vi "GUI_GlassmanEK40R15_VI.vi"() -> ()   [LabVIEW 2013]
uses:
  Shared/GUI_Template/GUI_master/tcp_new_data_event.ctl
  Shared/GUI_Template/GUI_master/tcp new data cluster.ctl
panel:
  out "tcp data event":T1
  in  "Refresh Button":bool
  in  "Select device":string(combo)="PL1-PresCtl"
  in  "stop":bool
  in  "enable::1":enum16{"off", "on", "reset", "fault"}(ring) caption="Enable HV"
  in  "voltage::1":dbl caption="Voltage (KV)" min=0.0 max=40.0
  out "voltageMode::1":enum16{"off", "on"}(ring) caption="Voltage Mode"
  in  "GUIdevice 1":string="PL1-GlassmanHV"
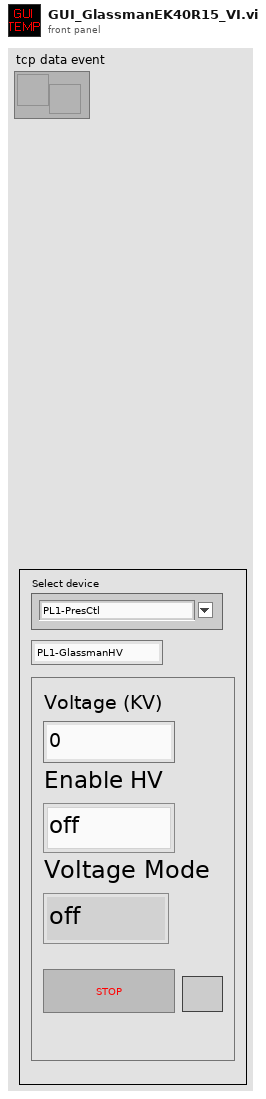
[diagram p1: front panel]
types:
  T1 = typedef "tcp_new_data_event.ctl" = refnum<user-event>
  T2 = enum32{"invalid app kind", "Development System", "Run Time System", "Student Edition", "Embedded LabVIEW", "Evaluation", "Custom"}
  T3 = typedef "tcp new data cluster.ctl" = cluster{"EventEnum":enum16{"new data", "connection status update"}, "Device name":string}
  T4 = enum32{"Invalid", "Standard", "Closed", "Hidden", "Minimized", "Maximized"}
  T5 = cluster{"Core":cluster{"Current VI Reference":refnum<vi>, "Close Panel on Exit?":bool}, "Your Boolean data":bool, "Your string data":string, "SuperGUI":cluster{"STOP queue":refnum<queue>, "SuperGUI ref":refnum<vi>}}
  T6 = cluster{"STOP queue":refnum<queue>, "SuperGUI ref":refnum<vi>}
  T7 = cluster{"Current VI Reference":refnum<vi>, "Close Panel on Exit?":bool}
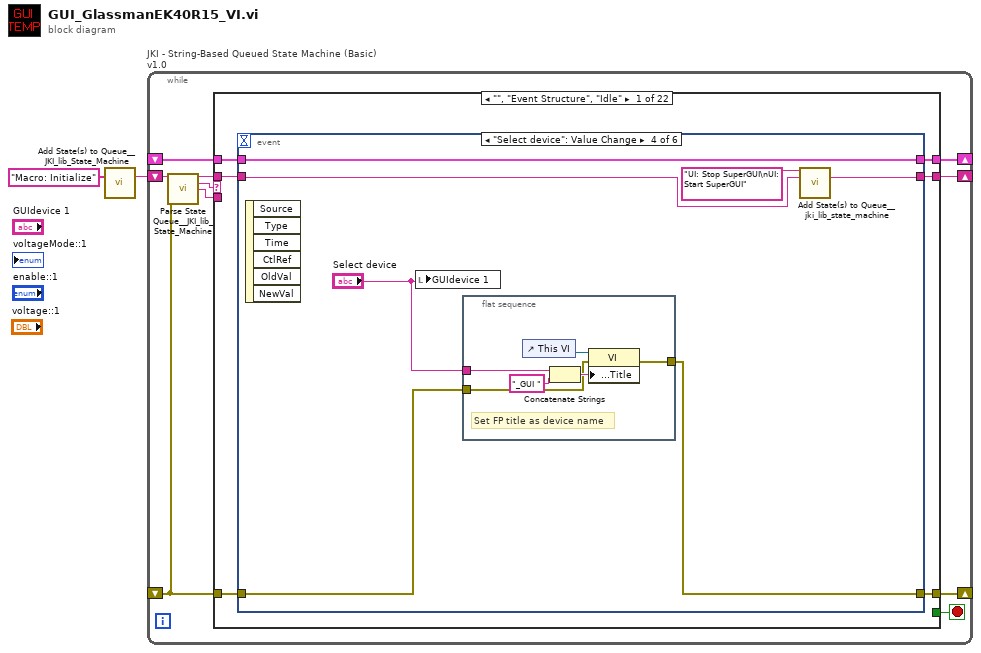
[diagram p0: block diagram]
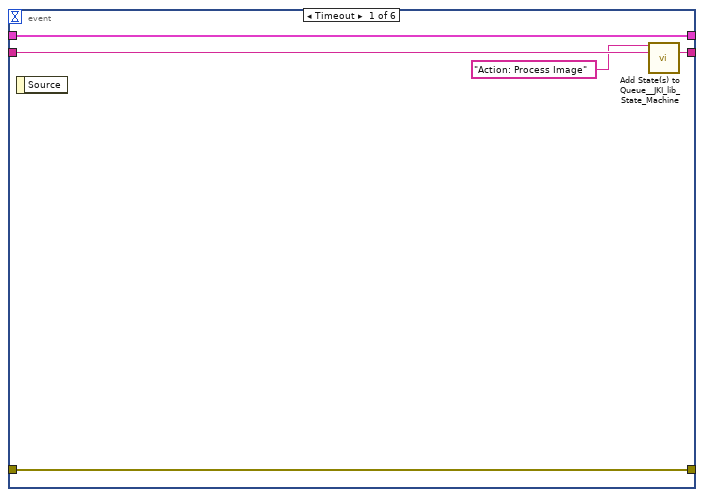
[diagram p2: hidden frame]
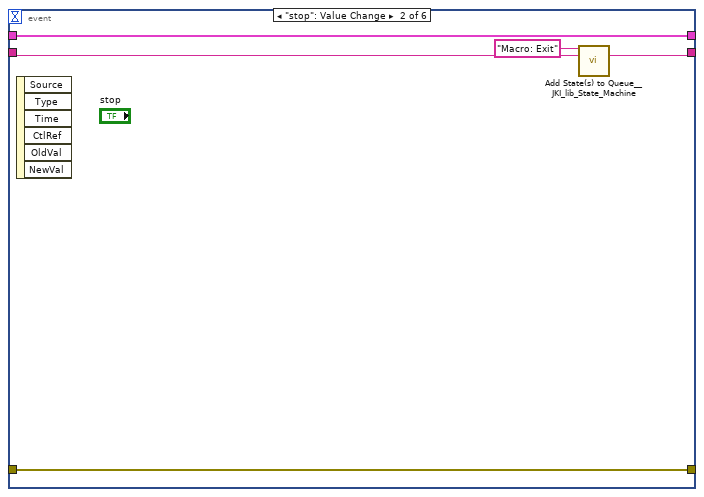
[diagram p3: hidden frame]
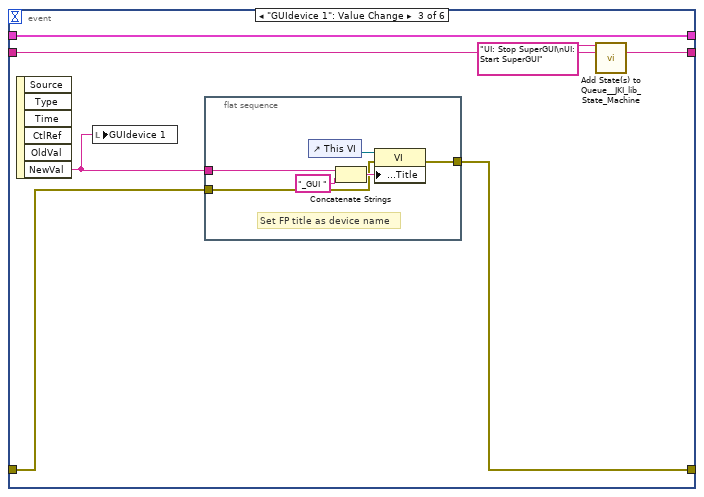
[diagram p4: hidden frame]
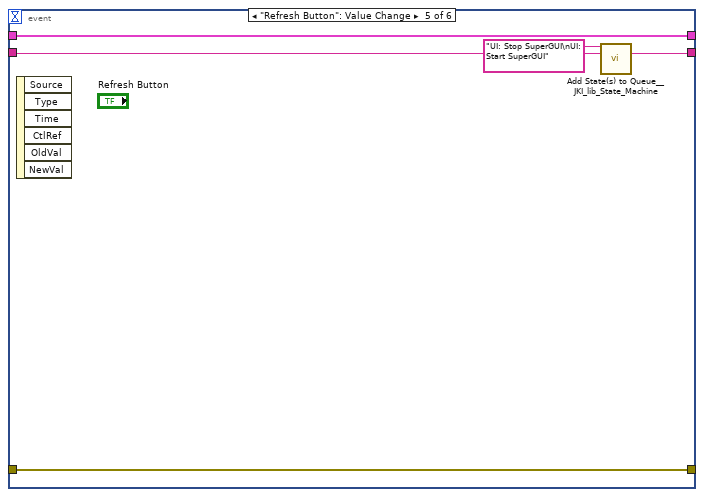
[diagram p5: hidden frame]
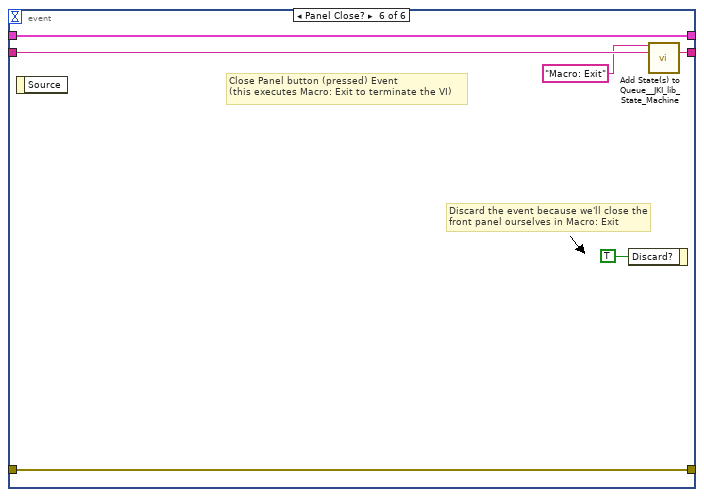
[diagram p6: hidden frame]
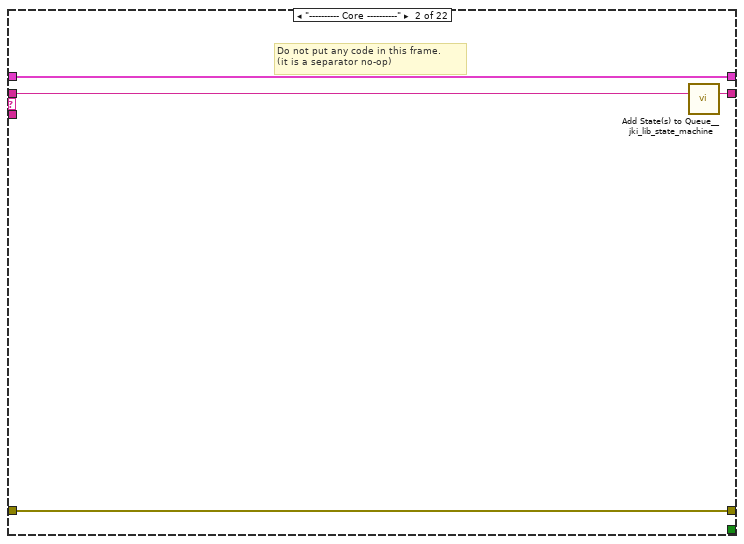
[diagram p7: hidden frame]
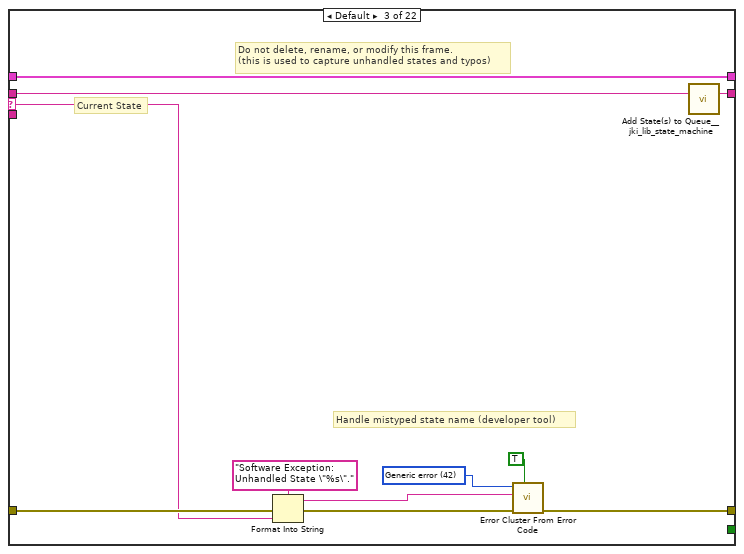
[diagram p8: hidden frame]
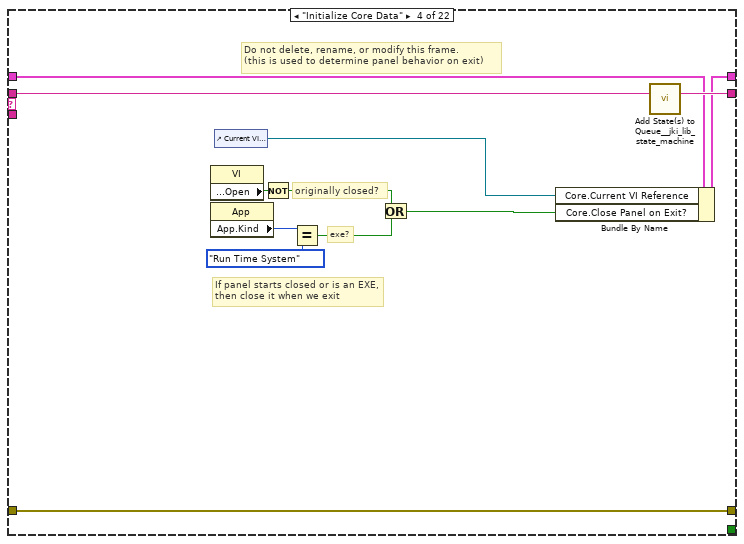
[diagram p9: hidden frame]
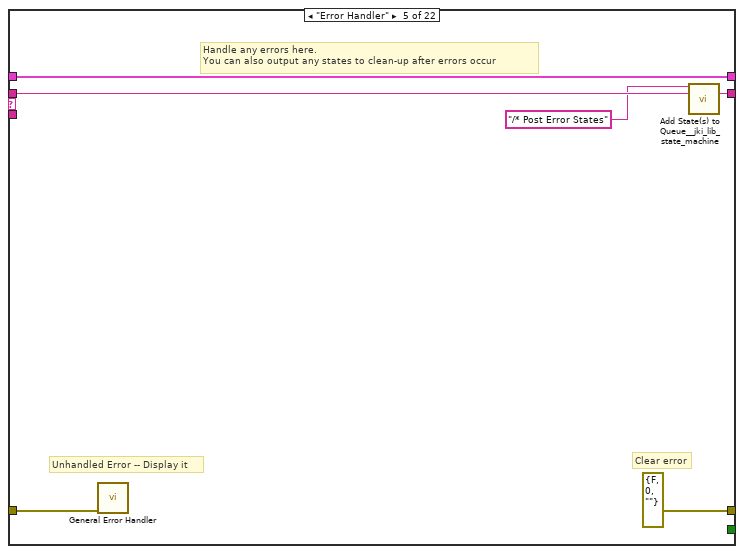
[diagram p10: hidden frame]
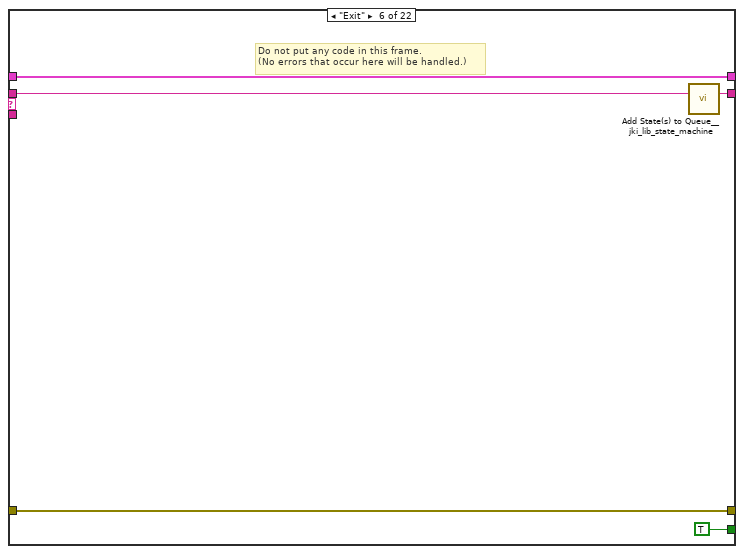
[diagram p11: hidden frame]
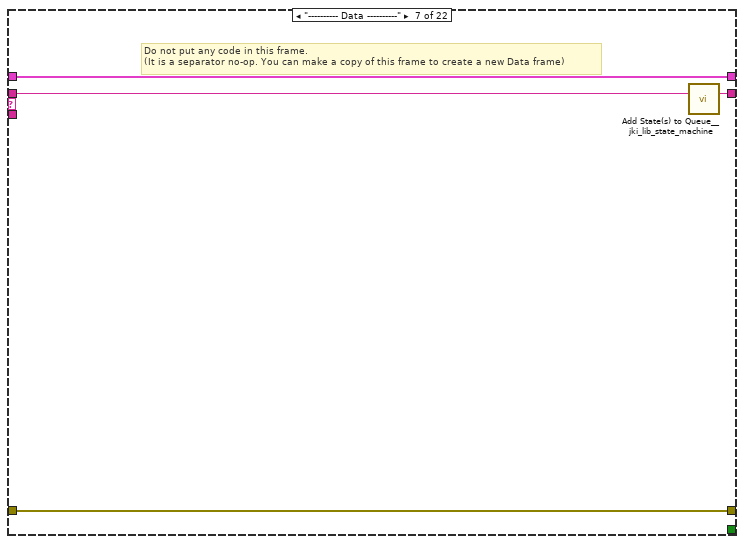
[diagram p12: hidden frame]
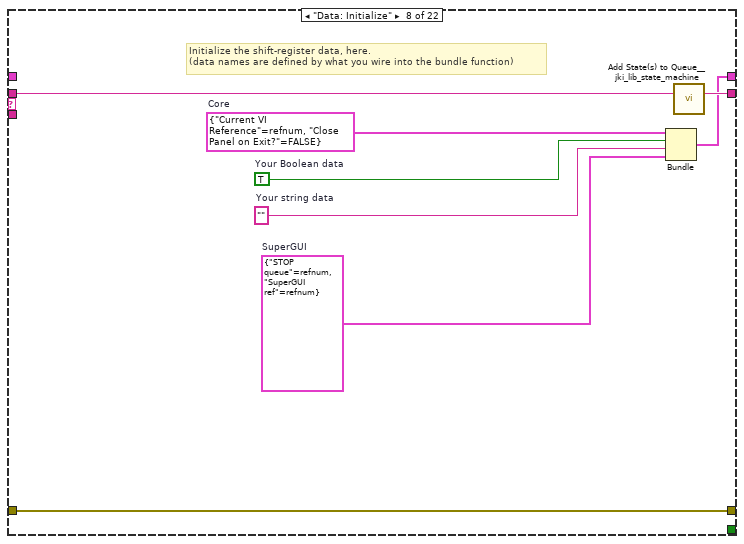
[diagram p13: hidden frame]
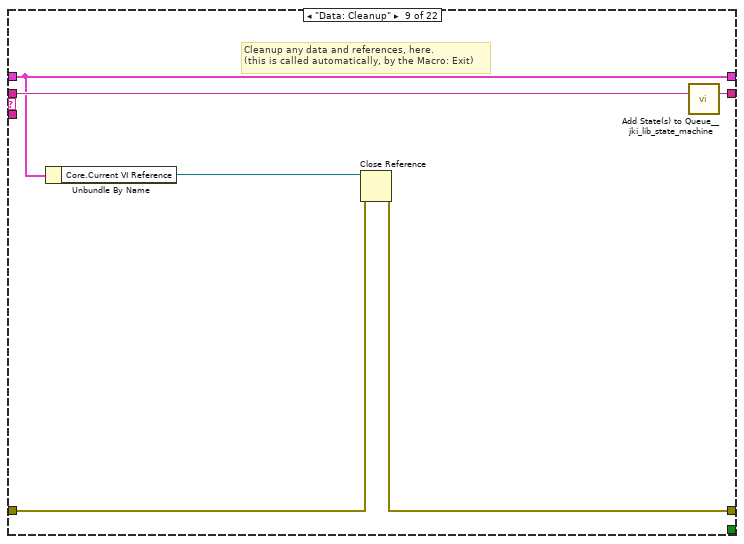
[diagram p14: hidden frame]
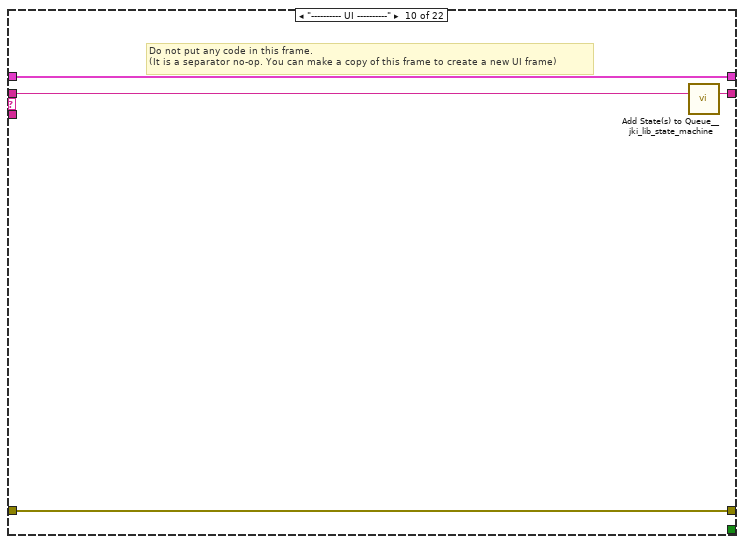
[diagram p15: hidden frame]
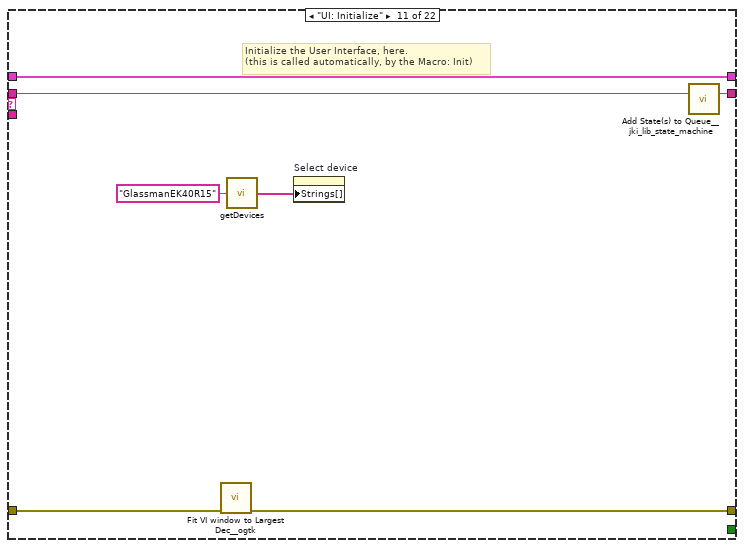
[diagram p16: hidden frame]
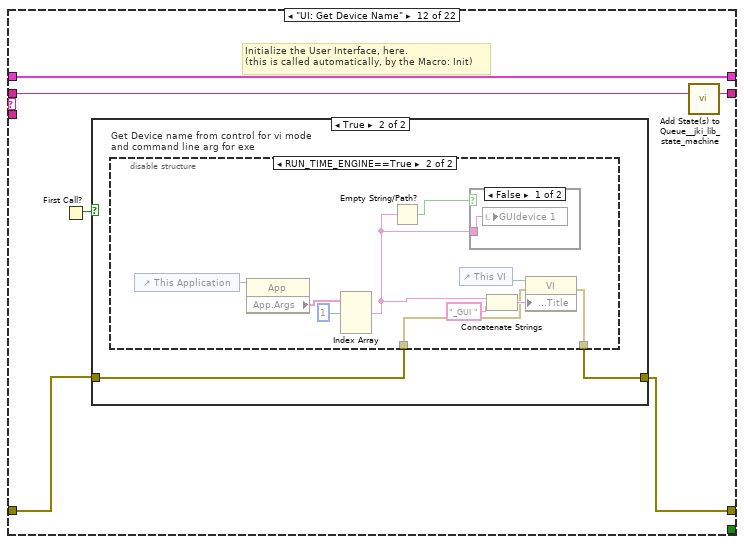
[diagram p17: hidden frame]
diagram:
  n1 = call <vilib>:"Add State(s) to Queue__JKI_lib_State_Machine.vi"("State(s) in (\"\")"="Macro: Initialize") -> ("States Out"=w2:string)  [unwired: 14 in]
  n2 = while "JKI - String-Based Queued State Machine (Basic) v1.0" {
    shift-right: [w5] -> _
    shift-left: _ -> [w4]
    shift-right: [w8] -> _
    shift-left: _ -> [w3]
    shift-right: [w7] -> _
    shift-left: w2 -> [w9]
    stop <- w6 stop-if-true
    n3 = call <vilib>:"Parse State Queue__JKI_lib_State_Machine.vi"("State Queue"=w9, "Error In (no error)"=w3) -> ("Remaining States"=w11:string, "Current State"=w12:string, "Arguments"=w10:string)  [unwired: 11 in]
    n4 = case shown="\"\", \"Event Structure\", \"Idle\"" w12 {
      selector: w12 -> [_ _ w70 _ _ _ _ _ _ _ _ _ _ _ _ _ _ _ _ _ _ _]
      tunnel: w11 -> [w18 w69 w74 w92 w98 w103 w107 w115 w121 w125 w132 w138 w173 w181 w187 w198 w224 w229 w239 w243 w247 w251]
      tunnel: w10 -> [_ _ _ _ _ _ _ _ _ _ _ _ _ _ w182 w192 _ _ _ _ _ _]
      tunnel: w4 -> [w16 w66 w72 w83 w95 w101 w104 _ w116 w122 w130 w136 w164 w176 w185 w194 w221 w226 w236 w240 w244 w248]
      tunnel: [w15 w67 w76 w89 errorcluster {"status"=FALSE, "code"=0, "source"=""} ("error out") w100 w105 w112 w117 w123 w128 w133 w157 w174 w183 w195 w222 w227 w237 w241 w245 w249] -> w8
      tunnel: w3 -> [w14 w67 w75 w89 w94 w100 w105 w112 w118 w123 w129 w134 w158 w175 w184 w196 w222 w227 w237 w241 w245 w249]
      tunnel: [w17 w68 w73 w91 w97 w102 w106 w114 w120 w124 w131 w137 w172 w180 w186 w197 w223 w228 w238 w242 w246 w250] -> w7
      tunnel: [_ _ _ _ _ TRUE _ _ _ _ _ _ _ _ _ _ _ _ _ _ _ _] -> w6
      tunnel: [w13 w66 w72 w90 w95 w101 w104 w113 w116 w122 w130 w136 w163 w176 w185 w194 w221 w226 w236 w240 w244 w248] -> w5
      frame "", "Event Structure", "Idle" {
        n5 = event shown="[3] \"Select device\": Value Change" {
          selector: _ -> [_ _ _ _ _ _]
          dyn-events: _ -> [_ _ _ _ _ _]
          timeout: _ -> [_ _ _ _ _ _]
          tunnel: w18 -> [w23 w26 w32 w43 w57 w65]
          tunnel: [w22 w25 w31 w42 w56 w64] -> w17
          tunnel: w16 -> [w20 w28 w35 w48 w59 w62]
          tunnel: [w21 w27 w33 w45 w58 w63] -> w15
          tunnel: w14 -> [w21 w27 w34 w46 w58 w63]
          tunnel: [w20 w28 w35 w48 w59 w62] -> w13
          event Timeout {
            n6 = event-data() -> ()  [unwired: 1 in, 1 out]
            n7 = call <vilib>:"Add State(s) to Queue__JKI_lib_State_Machine.vi"("State(s) in Front (\"\")"="Action: Process Image" ("State(s) in Front (\"\")"), "State(s) in (\"\")"=w23) -> ("States Out"=w22:string)  [unwired: 13 in]
          }
          event "stop": Value Change {
            n8 = event-data() -> ()  [unwired: 1 in, 6 out]
            n9 = call <vilib>:"Add State(s) to Queue__JKI_lib_State_Machine.vi"("State(s) in Front (\"\")"="Macro: Exit", "State(s) in (\"\")"=w26) -> ("States Out"=w25:string)  [unwired: 13 in]
          }
          event "GUIdevice 1": Value Change {
            n10 = event-data() -> ("NewVal"=w29:string)  [unwired: 1 in, 5 out]
            n11 = local write "GUIdevice 1"(w29) -> ()
            n12 = flat-sequence {
              tunnel: [w38] -> w33
              tunnel: w34 -> [w37]
              tunnel: w29 -> [w36]
              frame #0 {
                # "Set FP title as device name"
                n13 = control-ref of="This VI"() -> (w41:refnum<vi>)
                n14 = Concatenate Strings(w36, "_GUI ") -> (w40:string)
                n15 = property class="VI"(reference=w41, error in=w37, "Front Panel.Title"=w40) -> (error out=w38:errorcluster)  [unwired: 1 out]
              }
            }
            n16 = call <vilib>:"Add State(s) to Queue__JKI_lib_State_Machine.vi"("State(s) in Front (\"\")"="UI: Stop SuperGUI\nUI: Start SuperGUI", "State(s) in (\"\")"=w32) -> ("States Out"=w31:string)  [unwired: 13 in]
          }
          event "Select device": Value Change {
            n17 = event-data() -> ()  [unwired: 1 in, 6 out]
            n18 = local write "GUIdevice 1"("Select device") -> ()
            n19 = flat-sequence {
              tunnel: [w51] -> w45
              tunnel: w46 -> [w50]
              tunnel: "Select device" -> [w49]
              frame #0 {
                # "Set FP title as device name"
                n20 = control-ref of="This VI"() -> (w54:refnum<vi>)
                n21 = Concatenate Strings(w49, "_GUI ") -> (w53:string)
                n22 = property class="VI"(reference=w54, error in=w50, "Front Panel.Title"=w53) -> (error out=w51:errorcluster)  [unwired: 1 out]
              }
            }
            n23 = call <vilib>:"Add State(s) to Queue__jki_lib_state_machine.vi"("State(s) in Front (\"\")"="UI: Stop SuperGUI\nUI: Start SuperGUI", "State(s) in (\"\")"=w43) -> ("States Out"=w42:string)  [unwired: 13 in]
          }
          event "Refresh Button": Value Change {
            n24 = event-data() -> ()  [unwired: 1 in, 6 out]
            n25 = call <vilib>:"Add State(s) to Queue__JKI_lib_State_Machine.vi"("State(s) in Front (\"\")"="UI: Stop SuperGUI\nUI: Start SuperGUI", "State(s) in (\"\")"=w57) -> ("States Out"=w56:string)  [unwired: 13 in]
          }
          event Panel Close? {
            # "Discard the event because we'll close the front panel ourselves in Macro: Exit"
            # "Close Panel button (pressed) Event\n(this executes Macro: Exit to terminate the VI)"
            n26 = event-data() -> ()  [unwired: 1 in, 1 out]
            n27 = event-data("Discard?"=TRUE) -> ()  [unwired: 1 in, 1 out]
            n28 = call <vilib>:"Add State(s) to Queue__JKI_lib_State_Machine.vi"("State(s) in Front (\"\")"="Macro: Exit", "State(s) in (\"\")"=w65) -> ("States Out"=w64:string)  [unwired: 13 in]
          }
        }
      }
      frame "---------- Core ----------" {
        # "Do not put any code in this frame.\n(it is a separator no-op)"
        n29 = call <vilib>:"Add State(s) to Queue__jki_lib_state_machine.vi"("State(s) in (\"\")"=w69) -> ("States Out"=w68:string)  [unwired: 14 in]
      }
      frame Default {
        w79 = 42 items=["No error", "Argument error", "Memory is full", "Out of zone", "End of file", "File already open", "Generic file I/O error", "File not found", "File permission error", "Disk is full", "Duplicate path", "Too many files open", "System feature not enabled", "Resource file not found", "Cannot add resource", "Resource not found", "Image not found", "Image memory error", "Pen does not exist", "Config type invalid", "Config token not found", "Config parse error", "Config memory error", "Bad external code format", "Bad external code offset", "External code not present", "Null window", "Destroy window error", "Null menu", "Print aborted", "Bad print record", "Print driver error", "Windows error during printing", "Memory error during printing", "Print dialog error", "Generic print error", "Invalid device refnum", "Device not found", "Device parameter error", "Device unit error", "Cannot open device", "Device call aborted", "Generic error", "Cancelled by user", "Object ID too low", "Object ID too high", "Object not in heap", "Unknown heap", "Unknown object (invalid DefProc)", "Unknown object (DefProc not in table)", "Message out of range", "Invalid (null) method", "Unknown message", "Manager call not supported", "Bad address", "Network operation in progress", "Network operation timed out", "Connection is busy", "Network attribute not supported", "Network error", "Address in use", "System out of memory", "Connection aborted", "Connection refused", "Not connected", "Already connected", "Connection closed", "Initialization error (interapplication manager)", "Bad occurrence", "Wait on unbound occurrence handler", "Occurrence queue overflow", "Datalog type conflict", "Unused", "Unrecognized type (interapplication manager)", "Memory corrupt", "Failed to make temporary DLL", "Old CIN version", "Drag socket not found", "Failed to load drop-object", "Failed to register OLE object", "Failed to release OLE object", "Format specifier type mismatch", "Unknown format specifier", "Too few format specifiers", "Too many format specifiers", "Scan failed", "Newer CIN version", "Error converting to variant", "Runtime menu error", "Password tampered", "Variant attribute not found", "Incompatible variant data type", "Event data is not available", "Event Store is not present", "Occurrence is not found", "Event Queue is not created", "Event info is not available", "Refnum passed is NULL", "Error retrieving Class GUID", "Error retrieving CoClass GUID", "Error retrieving TypeLib GUID.", "Bad built application magic bytes.", "Specific driver is different from the specific driver associated with the Logical Name.", "There is no session opened to the class driver.", "Max Error", "MAX - Error with config objects", "MAX - Error loading configuration", "MAX - Group not supported"]
        # "Current State"
        # "Do not delete, rename, or modify this frame.\n(this is used to capture unhandled states and typos)"
        # "Handle mistyped state name (developer tool)"
        n30 = Format Into String(format string="Software Exception: Unhandled State \"%s\"." ("message"), error in=w75, w70) -> (resulting string=w78:string, error out=w77:errorcluster)  [unwired: 1 in]
        n31 = call <vilib>:"Error Cluster From Error Code.vi"("show call chain? (False)"=TRUE, "error in (no error)"=w77, "error message (\"\")"=w78, "error code (0)"=w79) -> ("error out"=w76:errorcluster)  [unwired: 5 in]
        n32 = call <vilib>:"Add State(s) to Queue__jki_lib_state_machine.vi"("State(s) in (\"\")"=w74) -> ("States Out"=w73:string)  [unwired: 14 in]
      }
      frame "Initialize Core Data" {
        # "Do not delete, rename, or modify this frame.\n(this is used to determine panel behavior on exit)"
        # "originally closed?"
        # "exe?"
        # "If panel starts closed or is an EXE, then close it when we exit"
        n33 = property class="VI"() -> ("Front Panel.Open"=w88:bool)  [unwired: 2 in, 2 out]
        n34 = property class="App"() -> ("App.Kind"=w87:T2)  [unwired: 2 in, 2 out]
        n35 = control-ref of="Current VI Reference"() -> (w81:refnum<vi>)
        n36 = Not(x=w88) -> (.not. x?=w85:bool)
        n37 = Equal?(x=w87, y=T2."Run Time System" ("Application:Kind")) -> (x = y?=w84:bool)
        n38 = Or(x=w85, y=w84) -> (x .or. y?=w82:bool)
        n39 = Bundle By Name(cluster=w83, "Core.Current VI Reference"=w81, "Core.Close Panel on Exit?"=w82) -> (w90:T5)
        n40 = call <vilib>:"Add State(s) to Queue__jki_lib_state_machine.vi"("State(s) in (\"\")"=w92) -> ("States Out"=w91:string)  [unwired: 14 in]
      }
      frame "Error Handler" {
        # "Unhandled Error -- Display it"
        # "Handle any errors here.\nYou can also output any states to clean-up after errors occur"
        # "Clear error"
        n41 = call <vilib>:"General Error Handler.vi"("error in (no error)"=w94) -> ()  [unwired: 10 in, 5 out]
        n42 = call <vilib>:"Add State(s) to Queue__jki_lib_state_machine.vi"("State(s) in Front (\"\")"="/* Post Error States", "State(s) in (\"\")"=w98) -> ("States Out"=w97:string)  [unwired: 13 in]
      }
      frame "Exit" {
        # "Do not put any code in this frame.\n(No errors that occur here will be handled.)"
        n43 = call <vilib>:"Add State(s) to Queue__jki_lib_state_machine.vi"("State(s) in (\"\")"=w103) -> ("States Out"=w102:string)  [unwired: 14 in]
      }
      frame "---------- Data ----------" {
        # "Do not put any code in this frame.\n(It is a separator no-op. You can make a copy of this frame to create a new Data frame)"
        n44 = call <vilib>:"Add State(s) to Queue__jki_lib_state_machine.vi"("State(s) in (\"\")"=w107) -> ("States Out"=w106:string)  [unwired: 14 in]
      }
      frame "Data: Initialize" {
        w108 = T6 {"STOP queue"=refnum, "SuperGUI ref"=refnum}  # SuperGUI
        w109 = T7 {"Current VI Reference"=refnum, "Close Panel on Exit?"=FALSE}  # Core
        w111 = TRUE  # Your Boolean data
        w110 = ""  # Your string data
        # "Initialize the shift-register data, here.\n(data names are defined by what you wire into the bundle function)"
        n45 = Bundle("Core"=w109, "Your Boolean data"=w111, "Your string data"=w110, "SuperGUI"=w108) -> (w113:T5)  [unwired: 1 in]
        n46 = call <vilib>:"Add State(s) to Queue__jki_lib_state_machine.vi"("State(s) in (\"\")"=w115) -> ("States Out"=w114:string)  [unwired: 14 in]
      }
      frame "Data: Cleanup" {
        # "Cleanup any data and references, here.\n(this is called automatically, by the Macro: Exit)"
        n47 = Unbundle By Name(w116) -> ("Core.Current VI Reference"=w119:refnum<vi>)
        n48 = Close Reference(reference=w119, error in (no error)=w118) -> (error out=w117:errorcluster)
        n49 = call <vilib>:"Add State(s) to Queue__jki_lib_state_machine.vi"("State(s) in (\"\")"=w121) -> ("States Out"=w120:string)  [unwired: 14 in]
      }
      frame "---------- UI ----------" {
        # "Do not put any code in this frame.\n(It is a separator no-op. You can make a copy of this frame to create a new UI frame)"
        n50 = call <vilib>:"Add State(s) to Queue__jki_lib_state_machine.vi"("State(s) in (\"\")"=w125) -> ("States Out"=w124:string)  [unwired: 14 in]
      }
      frame "UI: Initialize" {
        # "Initialize the User Interface, here.\n(this is called automatically, by the Macro: Init)"
        n51 = call <userlib>:"Fit VI window to Largest Dec__ogtk.vi"("error in (no error)"=w129) -> ("error out"=w128:errorcluster)  [unwired: 5 in, 1 out]
        n52 = call "getDevices.vi"("Device Class"="GlassmanEK40R15") -> ("All Devices"=w126:string[])
        n53 = property on="Select device" class="CmbBox"("Strings[]"=w126) -> ()  [unwired: 2 in, 2 out]
        n54 = call <vilib>:"Add State(s) to Queue__jki_lib_state_machine.vi"("State(s) in (\"\")"=w132) -> ("States Out"=w131:string)  [unwired: 14 in]
      }
      frame "UI: Get Device Name" {
        # "Initialize the User Interface, here.\n(this is called automatically, by the Macro: Init)"
        n55 = First Call?() -> (First Call?: T/F=w135:bool)
        n56 = case shown="True" w135 {
          tunnel: w134 -> [w139 w141]
          tunnel: [w139 w140] -> w133
          frame False {
          }
          frame True {
            n57 = disable-structure "Get Device name from control for vi mode\nand command line arg for exe" shown="RUN_TIME_ENGINE==True" {
              disable-tunnel: w141 -> [w142 w144]
              disable-tunnel: [w142 w143] -> w140
              frame condition #0 (active) {
              }
              frame condition #1 {
                n58 = control-ref of="This Application"() -> (w152:refnum<vi>)
                n59 = property class="App"(reference=w152) -> ("App.Args"=w151:string[])  [unwired: 1 in, 2 out]
                n60 = Index Array(array=w151, index #1=1 ("index")) -> (element #1=w145:string)  [unwired: 2 in, 2 out]
                n61 = Empty String/Path?(string/path=w145) -> (empty?=w149:bool)
                n62 = control-ref of="This VI"() -> (w148:refnum<vi>)
                n63 = case shown="False" w149 {
                  tunnel: w145 -> [w153 _]
                  frame False {
                    n64 = local write "GUIdevice 1"(w153) -> ()
                  }
                  frame True {
                  }
                }
                n65 = Concatenate Strings(w145, "_GUI ") -> (w147:string)
                n66 = property class="VI"(reference=w148, error in=w144, "Front Panel.Title"=w147) -> (error out=w143:errorcluster)  [unwired: 1 out]
              }
            }
          }
        }
        n67 = call <vilib>:"Add State(s) to Queue__jki_lib_state_machine.vi"("State(s) in (\"\")"=w138) -> ("States Out"=w137:string)  [unwired: 14 in]
      }
      frame "UI: Start SuperGUI" {
        # "create stop queue for supergui and its clones"
        # "x100 abort will be dependent on caller VI\nx80 abort will be independent of caller vi, this will abort vi when labview is closed."
        # "Start SuperGUI asynchronous way"
        n68 = vi-ref "GUI_Master_subvi_reentrant_queues.vi"() -> (w156:refnum<vi>)
        n69 = property class="VI"(reference=w156) -> ("Path"=w155:path)  [unwired: 1 in, 2 out]
        n70 = Create User Event(user event datatype=T3 {"EventEnum"=enum."new data", "Device name"="Device name"} ("New Event"), error in=w158) -> (user event=w159:refnum<user-event>, error out=w165:errorcluster)
        "tcp data event" <- w159
        n71 = control-ref of="This Application"() -> (w162:refnum<vi>)
        n72 = control-ref of="This VI"() -> (w161:refnum<vi>)
        n73 = Open VI Reference(type specifier VI Refnum (for type only)=refnum<vi> refnum, vi path=w155, options=256) -> (vi reference=w171:refnum<vi>, error out=w170:errorcluster)  [unwired: 3 in]
        n74 = register-events(w159) -> ()  [unwired: 2 in, 2 out]
        n75 = call "supergui create stop queue.vi"() -> ("STOP Queue out"=w167:refnum<queue>)  [unwired: 11 in]
        n76 = Current VI's Menubar() -> (w160:refnum<k9>)
        n77 = call-by-ref "Start Asynchronous Call"(reference=w171, error in=w170, "STOP Queue in"=w167, "This Application"=w162, 8:"error in (no error)"=w165, "tcp data event"=w159, "Caller menu reference"=w160, "Caller VI ref"=w161) -> (reference out=w154:refnum<vi>, error out=w157:errorcluster)  [unwired: 5 in, 1 out]
        n78 = Bundle By Name(cluster=w164, "SuperGUI.SuperGUI ref"=w154, "SuperGUI.STOP queue"=w167) -> (w163:T5)
        n79 = call <vilib>:"Add State(s) to Queue__jki_lib_state_machine.vi"("State(s) in (\"\")"=w173) -> ("States Out"=w172:string)  [unwired: 14 in]
      }
      frame "UI: Stop SuperGUI" {
        # "Stop Supergui Clone and wait until it exit properly"
        n80 = Unbundle By Name(w176) -> ("SuperGUI.SuperGUI ref"=w178:refnum<vi>, "SuperGUI.STOP queue"=w177:refnum<queue>)
        n81 = Release Queue(queue=w177, error in (no error)=w175) -> (error out=w179:errorcluster)  [unwired: 1 in, 2 out]
        n82 = call-by-ref "Wait On Asynchronous Call"(reference=w178, error in=w179) -> ("error out"=w174:errorcluster)  [unwired: 11 in, 2 out]
        n83 = call <vilib>:"Add State(s) to Queue__jki_lib_state_machine.vi"("State(s) in (\"\")"=w181) -> ("States Out"=w180:string)  [unwired: 14 in]
      }
      frame "UI: Cursor Set" {
        # "Argument"
        # "Set and Unset Cursor Busy.\n(Usage: \"UI: Cursor Set >> Busy|Idle\")"
        n84 = case shown="\"Idle\", Default" w182 {
          tunnel: w184 -> [w189 w191]
          tunnel: [w188 w190] -> w183
          frame "Idle", Default {
            n85 = call <vilib>:"Unset Busy.vi"("error in (no error)"=w189) -> ("error out"=w188:errorcluster)  [unwired: 10 in]
          }
          frame "Busy" {
            n86 = call <vilib>:"Set Busy.vi"("error in (no error)"=w191) -> ("error out"=w190:errorcluster)  [unwired: 9 in, 1 out]
          }
        }
        n87 = call <vilib>:"Add State(s) to Queue__jki_lib_state_machine.vi"("State(s) in (\"\")"=w187) -> ("States Out"=w186:string)  [unwired: 14 in]
      }
      frame "UI: Front Panel State" {
        # "Argument"
        # "Set Front Panel Open or Closed\n(Usage: \"UI: Front Panel State >> Open|Close\")"
        n88 = Unbundle By Name(w194) -> ("Core.Current VI Reference"=w193:refnum<vi>)
        n89 = case shown="\"Open\", Default" w192 {
          tunnel: w196 -> [w202 w215]
          tunnel: [w204 w216] -> w195
          tunnel: w193 -> [w203 w213]
          frame "Open", Default {
            n90 = property class="VI"(reference=w203, error in=w202) -> (reference out=w200:refnum<vi>, error out=w201:errorcluster, "Front Panel.Open"=w199:bool)
            n91 = case shown="False" w199 {
              tunnel: [w207 w210] -> w204
              tunnel: w201 -> [w206 w210]
              tunnel: w200 -> [w205 _]
              frame False {
                n92 = invoke class="VI" method="FP.Open"(reference=w205, error in=w206, "Activate"=TRUE, "State"=T4."Standard") -> (error out=w207:errorcluster)  [unwired: 1 in, 4 out]
              }
              frame True {
              }
            }
          }
          frame "Close" {
            n93 = property class="VI"(reference=w213, error in=w215) -> (reference out=w212:refnum<vi>, error out=w214:errorcluster, "Front Panel.Open"=w211:bool)
            n94 = case shown="True" w211 {
              tunnel: [w217 w220] -> w216
              tunnel: w214 -> [w217 w219]
              tunnel: w212 -> [_ w218]
              frame False {
              }
              frame True {
                n95 = invoke class="VI" method="FP.Close"(reference=w218, error in=w219) -> (error out=w220:errorcluster)  [unwired: 1 in, 2 out]
              }
            }
          }
        }
        n96 = call <vilib>:"Add State(s) to Queue__jki_lib_state_machine.vi"("State(s) in (\"\")"=w198) -> ("States Out"=w197:string)  [unwired: 14 in]
      }
      frame "---------- Macro ----------" {
        # "Do not put any code in this frame.\n(It is a separator no-op. You can make a copy of this frame to create a new Macro frame)"
        n97 = call <vilib>:"Add State(s) to Queue__jki_lib_state_machine.vi"("State(s) in (\"\")"=w224) -> ("States Out"=w223:string)  [unwired: 14 in]
      }
      frame "Macro: Initialize" {
        # "Initialization Macro\n(This is called once, when the VI starts)"
        n98 = call <vilib>:"Add State(s) to Queue__jki_lib_state_machine.vi"("State(s) in Front (\"\")"="Data: Initialize\nInitialize Core Data\nUI: Initialize\nUI: Get Device Name\nUI: Start SuperGUI\nUI: Front Panel State >> Open", "State(s) in (\"\")"=w229) -> ("States Out"=w228:string)  [unwired: 13 in]
      }
      frame "Macro: Exit" {
        # "Exit Macro\n(This is called once, when the VI exits)"
        n99 = Unbundle By Name(w236) -> ("Core.Close Panel on Exit?"=w235:bool)
        n100 = Select(t="UI: Front Panel State >> Close", s=w235, f="") -> (s? t:f=w232:string)
        n101 = call <vilib>:"Add State(s) to Queue__jki_lib_state_machine.vi"("State(s) in (\"\")"=w232, "State(s) at Back (\"\")"="Data: Cleanup\nExit") -> ("States Out"=w230:string)  [unwired: 13 in]
        n102 = call <vilib>:"Add State(s) to Queue__jki_lib_state_machine.vi"("State(s) in Front (\"\")"=w230, "State(s) in (\"\")"=w239) -> ("States Out"=w238:string)  [unwired: 13 in]
      }
      frame "---------- New Category ----------" {
        # "Template Separator\n(You can make a copy of, or modify, this frame)"
        n103 = call <vilib>:"Add State(s) to Queue__jki_lib_state_machine.vi"("State(s) in (\"\")"=w243) -> ("States Out"=w242:string)  [unwired: 14 in]
      }
      frame "New Category: 1" {
        # "Your code here.\n(You can make a copy of, or modify, this frame)"
        n104 = call <vilib>:"Add State(s) to Queue__jki_lib_state_machine.vi"("State(s) in (\"\")"=w247) -> ("States Out"=w246:string)  [unwired: 14 in]
      }
      frame "New Category: 2" {
        # "Your code here.\n(You can make a copy of, or modify, this frame)"
        n105 = call <vilib>:"Add State(s) to Queue__jki_lib_state_machine.vi"("State(s) in (\"\")"=w251) -> ("States Out"=w250:string)  [unwired: 14 in]
      }
    }
  }
